vi "myRIO Basic Read.vi"() -> ()   [LabVIEW 2014]
panel:
  in  "Timeout (ms) (-1: no timeout)":i32=10000
  in  "stop":bool
  in  "error in (no error)":errorcluster
  out "Characters Read":string
  in  "Character Count":u32=1
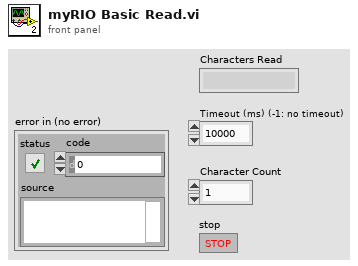
[diagram p1: front panel]
types:
  T1 = cluster{"Invert Polarity?":bool, "baud rate (9600)":u32, "data bits (8)":u16, "parity (0:none)":u16, "stop bits (10: 1 bit)":u16}
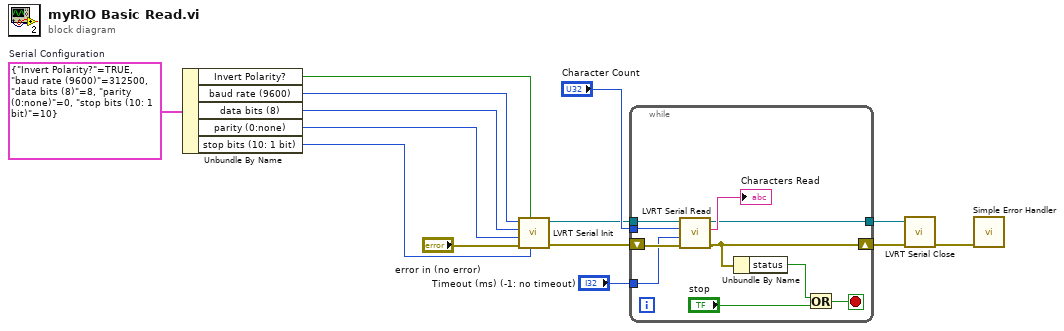
[diagram p0: block diagram]
diagram:
  w14 = T1 {"Invert Polarity?"=TRUE, "baud rate (9600)"=312500, "data bits (8)"=8, "parity (0:none)"=0, "stop bits (10: 1 bit)"=10}  # Serial Configuration
  n1 = Unbundle By Name(w14) -> ("Invert Polarity?"=w6:bool, "baud rate (9600)"=w11:u32, "data bits (8)"=w10:u16, "parity (0:none)"=w9:u16, "stop bits (10: 1 bit)"=w8:u16)
  n2 = call "LVRT Serial Init.vi"("stop bits (10: 1 bit)"=w8, "Invert Polarity?"=w6, "error in (no error)"="error in (no error)", "parity (0:none)"=w9, "data bits (8)"=w10, "baud rate (9600)"=w11) -> ("error out"=w4:errorcluster, "FPGA Main Reference Out"=w5:refnum<k20>)  [unwired: 4 in]
  n3 = while {
    shift-right: [w18] -> w12
    shift-left: w4 -> [w19]
    tunnel: "Character Count" -> [w20]
    tunnel: w5 -> [w21]
    tunnel: [w16] -> w2
    tunnel: "Timeout (ms) (-1: no timeout)" -> [w15]
    stop <- w24 stop-if-true
    n4 = call "LVRT Serial Read.vi"("error in (no error)"=w19, "Timeout (ms) (-1: no timeout)"=w15, "Bytes to Read"=w20, "FPGA Main Ref"=w21) -> ("error out"=w18:errorcluster, "String"=→"Characters Read":string, "FPGA Main Ref Out"=w16:refnum<k20>)  [unwired: 1 in, 4 out]
    n5 = Unbundle By Name(w18) -> ("status"=w23:bool)
    n6 = Or(x=w23, y="stop") -> (x .or. y?=w24:bool)
  }
  n7 = call "LVRT Serial Close.vi"("error out"=w12, "FPGA Main Ref"=w2) -> ("error out"=w3:errorcluster)  [unwired: 9 in]
  n8 = call <vilib>:"Simple Error Handler.vi"("error in (no error)"=w3) -> ()  [unwired: 4 in, 5 out]
